vi "EmsaMain.vi"() -> ()   [LabVIEW 2017]
uses:
  <vilib>/addons/InsightCM/Devices/Shared/Common/Trigger/Trigger.lvlib
  <vilib>/addons/InsightCM/Devices/Shared/Emsa/EmsaFPGABifileManager/EmsaFPGABitfileManager.lvlib
  <vilib>/addons/InsightCM/Devices/Shared/Emsa/EmsaAcquisition/EmsaAcquisition.lvlib
  <vilib>/addons/InsightCM/Devices/Shared/Emsa/EmsaAnalysis/EmsaAnalysis.lvlib
  <vilib>/addons/InsightCM/Devices/Shared/Emsa/EmsaDataFlowManager/EmsaDataFlowManager.lvlib
  <vilib>/addons/InsightCM/Devices/Shared/Emsa/EmsaAudio/EmsaAudio.lvlib
  <vilib>/addons/TraceLogger/TraceLogger.lvlib
  <vilib>/addons/TimerProcess/TimerProcess.lvlib
  <vilib>/addons/InsightCM/Devices/Shared/Common/Controller/Controller.lvlib
  <vilib>/addons/InsightCM/Devices/Shared/Common/ServerComm/ServerComm.lvlib
  <vilib>/addons/BlinkProcess/BlinkProcess.lvlib
  <vilib>/addons/InsightCM/Devices/Shared/Common/FileManager/FileManager.lvlib
  <vilib>/addons/InsightCM/Devices/Shared/Common/TracePointDisplay/TracePointDisplay.lvlib
  <vilib>/addons/InsightCM/Devices/Shared/Common/TrendAlarm/TrendAlarm.lvlib
  <vilib>/addons/WatchdogProcess/WatchdogProcess.lvlib
  <vilib>/addons/InsightCM/Utilities/GlobalConfiguration/GlobalConfiguration.lvlib
  <vilib>/addons/InsightCM/Utilities/PropertyHelpers/PropertyHelpers.lvlib
  <vilib>/addons/InsightCM/Devices/Shared/Common/OpState/OpState.lvlib
  <vilib>/addons/InsightCM/Devices/Shared/Emsa/EmsaDataEventCreator/EmsaDataEventCreator.lvlib
  <vilib>/addons/InsightCM/Devices/Shared/Common/DeviceHealth/DeviceHealth.lvlib
  <vilib>/addons/InsightCM/Devices/Shared/Emsa/EmsaTestPanel/EmsaTestPanel.lvlib
panel:
  out "debug":string
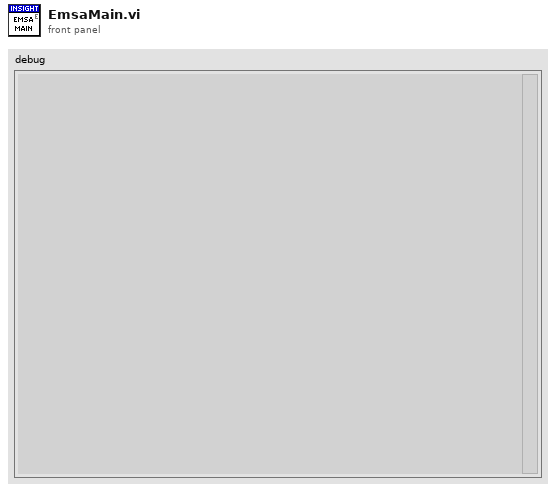
[diagram p1: front panel]
types:
  T1 = typedef "SectionKeyValues.ctl" = cluster{"Section":string, "KeyValues":T2[]}
  T2 = typedef "KeyValuePair.ctl" = cluster{"Key":string, "Value":string}
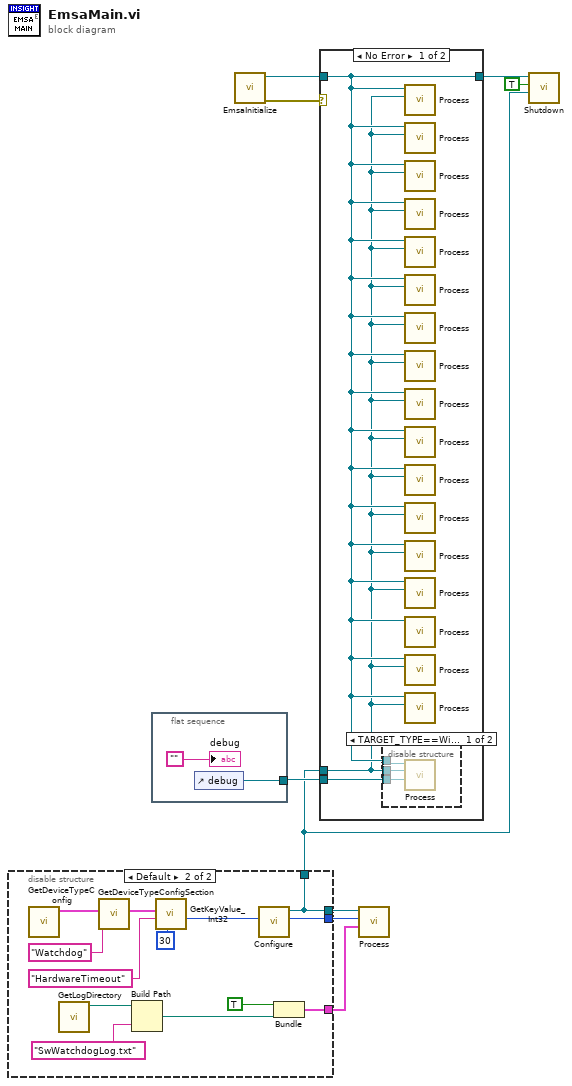
[diagram p0: block diagram]
diagram:
  n1 = disable-structure shown="Default" {
    disable-tunnel: [_ w22] -> w4
    disable-tunnel: [_ w22] -> w3
    disable-tunnel: [_ w21] -> w2
    disable-tunnel: [_ w11] -> w1
    frame condition #0 {
    }
    frame condition #1 (active) {
      n2 = call <vilib>:"GetDeviceTypeConfig.vi"() -> ("key values"=w16:T1[])  [unwired: 9 in, 2 out]
      n3 = call <vilib>:"GetLogDirectory.vi"() -> ("log dir"=w15:path)  [unwired: 10 in, 1 out]
      n4 = call <vilib>:"GetDeviceTypeConfigSection.vi"("key"="Watchdog", "key values"=w16) -> ("key value pairs out"=w19:T2[])  [unwired: 8 in, 1 out]
      n5 = Build Path(base path=w15, name or relative path="SwWatchdogLog.txt") -> (appended path=w13:path)
      n6 = call <vilib>:"GetKeyValue_Int32.vi"("default"=30, "key"="HardwareTimeout" ("Tag"), "key value pairs"=w19) -> ("value"=w10:i32)  [unwired: 6 in, 2 out]
      n7 = call <vilib>:"Configure.vi"("hw timeout (sec)"=w10) -> ("watchdogID out"=w21:u64, "Pound"=w22:refnum<class "Pound.lvclass">)  [unwired: 8 in, 1 out]
      n8 = Bundle(TRUE, "appended path"=w13) -> (w11:cluster{bool, "appended path":path})  [unwired: 1 in]
    }
  }
  n9 = flat-sequence {
    tunnel: [w23] -> w7
    frame #0 {
      n10 = control-ref of="debug"() -> (w23:refnum<vi>)
      "debug" <- ""
    }
  }
  n11 = call <vilib>:"EmsaInitialize.vi"() -> ("error out"=w9:errorcluster, "Qbus out"=w6:refnum<class "Qbus.lvclass">)  [unwired: 10 in]
  n12 = case shown="No Error" w9 {
    tunnel: w6 -> [w26 w31]
    tunnel: [w26 w31] -> w8
    tunnel: w4 -> [w25 _]
    tunnel: w7 -> [w27 _]
    frame No Error {
      n13 = disable-structure shown="TARGET_TYPE==Windows" {
        disable-tunnel: w27 -> [w30 _]
        disable-tunnel: w26 -> [w29 _]
        disable-tunnel: w25 -> [w28 _]
        frame condition #0 {
          n14 = call <vilib>:"Process.vi"("string refnum"=w30, "Pound in"=w28, "Qbus in"=w29) -> ()  [unwired: 8 in, 1 out]
        }
        frame condition #1 (active) {
        }
      }
      n15 = call <vilib>:"Process.vi"("Pound in"=w25, "Qbus in"=w26) -> ()  [unwired: 9 in, 1 out]
      n16 = call <vilib>:"Process.vi"("Pound in"=w25, "Qbus in"=w26) -> ()  [unwired: 9 in, 1 out]
      n17 = call <vilib>:"Process.vi"("Pound in"=w25, "Qbus in"=w26) -> ()  [unwired: 9 in, 1 out]
      n18 = call <vilib>:"Process.vi"("Pound in"=w25, "Qbus in"=w26) -> ()  [unwired: 9 in, 1 out]
      n19 = call <vilib>:"Process.vi"("Pound in"=w25, "Qbus in"=w26) -> ()  [unwired: 9 in, 1 out]
      n20 = call <vilib>:"Process.vi"("Pound in"=w25, "Qbus in"=w26) -> ()  [unwired: 9 in, 1 out]
      n21 = call <vilib>:"Process.vi"("Pound in"=w25, "Qbus in"=w26) -> ()  [unwired: 9 in, 1 out]
      n22 = call <vilib>:"Process.vi"("Pound in"=w25, "Qbus in"=w26) -> ()  [unwired: 9 in, 1 out]
      n23 = call <vilib>:"Process.vi"("Pound in"=w25, "Qbus in"=w26) -> ()  [unwired: 9 in, 1 out]
      n24 = call <vilib>:"Process.vi"("Pound in"=w25, "Qbus in"=w26) -> ()  [unwired: 9 in, 1 out]
      n25 = call <vilib>:"Process.vi"("Pound in"=w25, "Qbus in"=w26) -> ()  [unwired: 9 in, 1 out]
      n26 = call <vilib>:"Process.vi"("Pound in"=w25, "Qbus in"=w26) -> ()  [unwired: 9 in, 1 out]
      n27 = call <vilib>:"Process.vi"("Pound in"=w25, "Qbus in"=w26) -> ()  [unwired: 9 in, 1 out]
      n28 = call <vilib>:"Process.vi"("Pound in"=w25, "Qbus in"=w26) -> ()  [unwired: 9 in, 1 out]
      n29 = call <vilib>:"Process.vi"("qbus in"=w26) -> ()  [unwired: 10 in, 1 out]
      n30 = call <vilib>:"Process.vi"("Pound"=w25, "Qbus in"=w26) -> ()  [unwired: 9 in, 1 out]
      n31 = call <vilib>:"Process.vi"("pound in"=w25, "qbus in"=w26) -> ()  [unwired: 9 in, 1 out]
    }
    frame Error {
    }
  }
  n32 = call <vilib>:"Process.vi"("Logging"=w1, "watchdogID"=w2, "Pound"=w3) -> ()  [unwired: 6 in, 3 out]
  n33 = call <vilib>:"Shutdown.vi"("Pound"=w4, "restart system"=TRUE, "Qbus in"=w8) -> ()  [unwired: 8 in, 1 out]
